vi "Unpack for gRPC.vi"(8 "error in":errorcluster, 9 "configuration / results":enum16{"Configuration", "Results"}(ring), 10 "any":T1, 11 "measurement plugin in":refnum<class "WorkflowDO.lvclass">) -> (0 "error out":errorcluster, 2 "data value":variant, 3 "measurement plugin out":refnum<class "WorkflowDO.lvclass">)   [LabVIEW 2025, in "WorkflowDO.lvclass"]
uses:
  WorkflowDO.lvclass
  <vilib>/gRPC/LabVIEW gRPC Library/Shared/Any.ctl
  Measurement Configuration.ctl
  Measurement Results.ctl
  a521b266-ce99-437c-923d-067dcf1e07fd.vi
  3ecd018e-d556-4cbc-bc60-c4ba57204520.vi
  <vilib>/gRPC/LabVIEW gRPC Library/Server API/Translate Protobuf Error.vi
  <vilib>/AdvancedString/1D String Array to Delimited String.vi
  <vilib>/gRPC/LabVIEW gRPC Library/Server API/Server/Get Server DLL Path.vi
  WorkflowDO.lvclass/WorkflowDO.ctl
  <vilib>/Plug-In SDKs/Measurements/Measurement Plugin Service/Measurement Plugin Service.lvclass
  <vilib>/gRPC/LabVIEW gRPC Library/grpc-lvsupport-release.lvlib
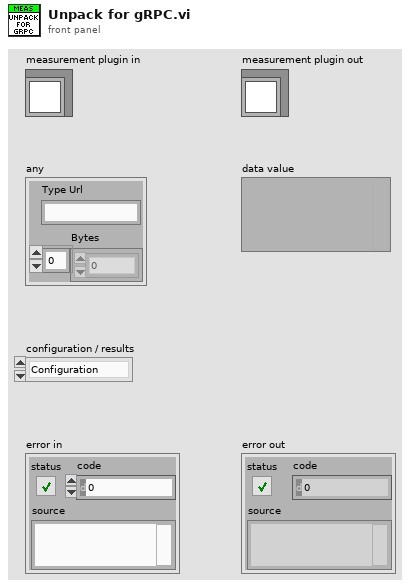
[diagram p1: front panel]
types:
  T1 = typedef "grpc-lvsupport-release.lvlib/Any.ctl" = cluster{"Type Url":string, "Bytes":u8[]}
  T2 = typedef "grpc-lvsupport-release.lvlib/grpcId.ctl" = u64
  T3 = typedef "WorkflowDO.lvclass/Measurement Configuration.ctl" = cluster{"Counter":tag, "Output Terminal":tag, "Frequency":dbl, "Duty Cycle":dbl, "Number of Pulses":i32}
  T4 = typedef "WorkflowDO.lvclass/Measurement Results.ctl" = cluster{"Actual Frequency":dbl, "Actual Duty Cycle":dbl}
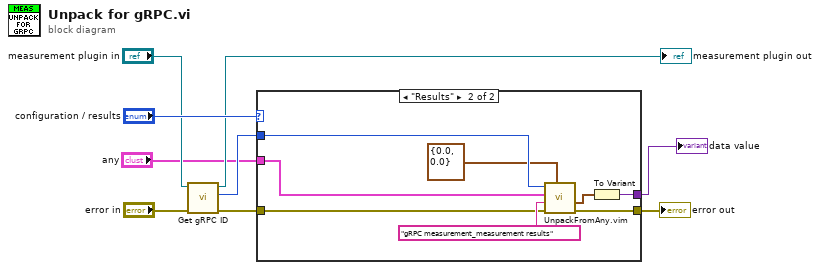
[diagram p0: block diagram]
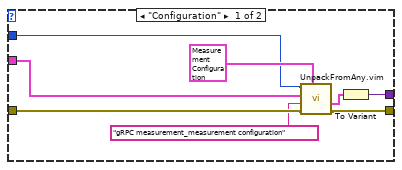
[diagram p2: hidden frame]
diagram:
  n1 = call <vilib>:"Get gRPC ID.vi"("error in"="error in", "measurement plugin service in"="measurement plugin in") -> ("error out"=w6:errorcluster, "gRPC ID"=w3:T2, "measurement plugin service out"=→"measurement plugin out":refnum<class "WorkflowDO.lvclass">)  [unwired: 7 in]
  n2 = case shown="\"Results\"" "configuration / results" {
    tunnel: w6 -> [w15 w19]
    tunnel: "any" -> [w10 w18]
    tunnel: w3 -> [w12 w22]
    tunnel: [w16 w23] -> w9
    tunnel: [w17 w25] -> w1
    frame "Configuration" {
      n3 = call "UnpackFromAny.vim"("Data Type"=T3 {"Counter"="Lorem ipsum dolor sit", "Output Terminal"="/Dev1/PFI12", "Frequency"=1.2, "Duty Cycle"=32.0, "Number of Pulses"=-32} ("Measurement Configuration"), "error in"=w15, "Message Type"="gRPC measurement_measurement configuration", "Any"=w10, "gRPCid in"=w12) -> ("error out"=w16:errorcluster, "Unpacked Value"=w14:T3)  [unwired: 4 in, 1 out]
      n4 = To Variant(anything=w14) -> (Variant=w17:variant)
    }
    frame "Results" {
      n5 = call "UnpackFromAny.vim"("Data Type"=T4 {"Actual Frequency"=0.0, "Actual Duty Cycle"=0.0} ("Measurement Results"), "error in"=w19, "Message Type"="gRPC measurement_measurement results", "Any"=w18, "gRPCid in"=w22) -> ("error out"=w23:errorcluster, "Unpacked Value"=w24:T4)  [unwired: 4 in, 1 out]
      n6 = To Variant(anything=w24) -> (Variant=w25:variant)
    }
  }
  "error out" <- w9
  "data value" <- w1
